vi "TBS2000Series_Init.vi"(0 "object in":refnum<class "TBS2000Series.lvclass">, 3 "VISA resource name":refnum<visa-resource-name>, 5 "error in (no error)":errorcluster) -> (14 "object out":refnum<class "TBS2000Series.lvclass">, 19 "error out":errorcluster)   [LabVIEW 2023, in "TBS2000Series.lvclass"]
uses:
  TBS2000Series.lvclass
  TBS2000Series.lvclass/TBS2000Series.ctl
  <instrlib>/Tektronix TBS 2000 Series/Tektronix TBS 2000 Series.lvlib
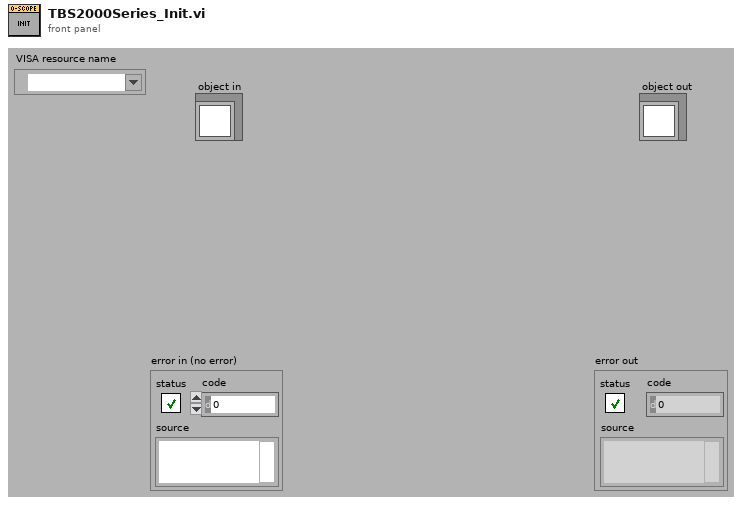
[diagram p1: front panel]
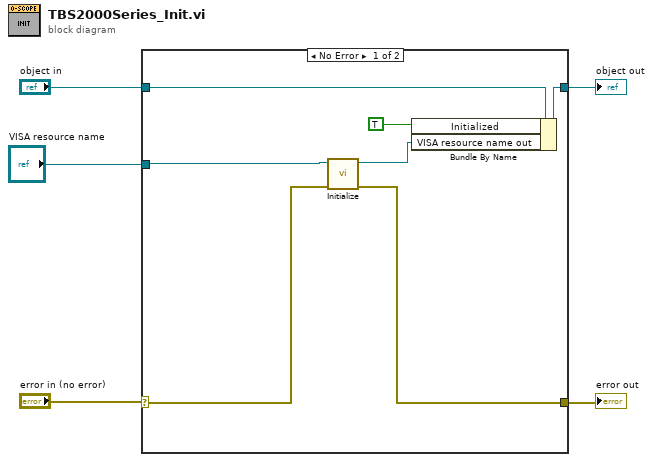
[diagram p0: block diagram]
diagram:
  n1 = case shown="No Error" "error in (no error)" {
    selector: "error in (no error)" -> [w12 w13]
    tunnel: "object in" -> [w9 w14]
    tunnel: [w8 w14] -> w4
    tunnel: [w11 w13] -> w2
    tunnel: "VISA resource name" -> [w10 _]
    frame No Error {
      n2 = call <instrlib>:"Initialize.vi"("error in (no error)"=w12, "VISA resource name"=w10) -> ("error out"=w11:errorcluster, "VISA resource name out"=w6:refnum<visa-resource-name>)  [unwired: 8 in]
      n3 = Bundle By Name(cluster=w9, "Initialized"=TRUE, "VISA resource name out"=w6) -> (w8:refnum<class "TBS2000Series.lvclass">)
    }
    frame Error {
    }
  }
  "object out" <- w4
  "error out" <- w2
